vi "SetControlSource.vi"(8 "error in (no error)":errorcluster, 11 "Laser Diode Controller in":refnum<class "KLD101.lvclass">) -> (0 "error out":errorcluster, 3 "Laser Diode Controller out":refnum<class "KLD101.lvclass">)   [LabVIEW 2016, in "Laser Diode Controller.lvlib" / "KLD101.lvclass"]
uses:
  KLD101.lvclass
  KLD101.lvclass/KLD101.ctl
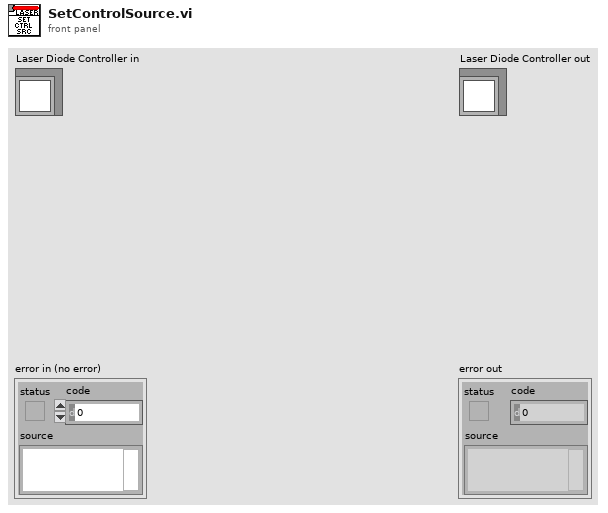
[diagram p1: front panel]
types:
  T1 = enum16{"Software Only", "External Signal", "Potentiometer"}
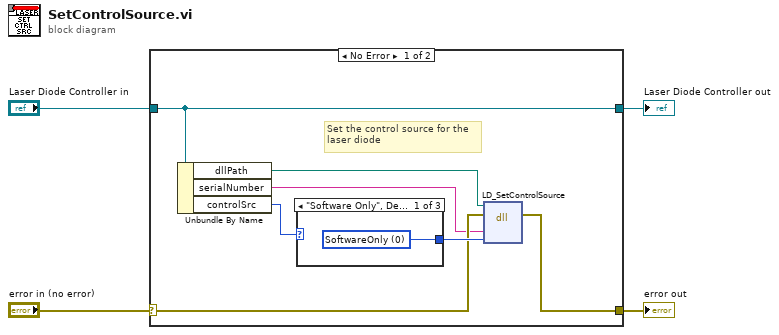
[diagram p0: block diagram]
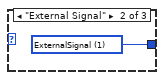
[diagram p2: hidden frame]
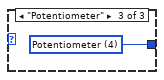
[diagram p3: hidden frame]
diagram:
  n1 = case shown="No Error" "error in (no error)" {
    selector: "error in (no error)" -> [w8 w16]
    tunnel: [w7 w16] -> w3
    tunnel: [w11 w15] -> w1
    tunnel: "Laser Diode Controller in" -> [w11 w15]
    frame No Error {
      # "Set the control source for the\nlaser diode"
      n2 = Unbundle By Name(w11) -> ("dllPath"=w5:path, "serialNumber"=w6:string, "controlSrc"=w10:T1)
      n3 = case shown="\"Software Only\", Default" w10 {
        tunnel: [w12 w13 w14] -> w9
        frame "Software Only", Default {
          w12 = u16 0 items=["SoftwareOnly"=0, "ExternalSignal"=1, "Potentiometer"=4] ("inputSource")
        }
        frame "External Signal" {
          w13 = u16 1 items=["SoftwareOnly"=0, "ExternalSignal"=1, "Potentiometer"=4] ("inputSource")
        }
        frame "Potentiometer" {
          w14 = u16 4 items=["SoftwareOnly"=0, "ExternalSignal"=1, "Potentiometer"=4] ("inputSource")
        }
      }
      n4 = dll-call lib="C:/IDEXX Software/Collimation/data/Thorlabs.MotionControl.KCube.LaserDiode.dll" fn="LD_SetControlSource"(path in=w5, error in=w8, "SerialNumber"=w6, "Source"=w9) -> (error out=w7:errorcluster)  [unwired: 4 in, 1 out]
    }
    frame Error {
    }
  }
  "error out" <- w3
  "Laser Diode Controller out" <- w1
